vi "SV Compare Signal Configurations.vi"(5 "SV Signal 1":refnum<class "SV Signal.lvclass">, 9 "SV Signal 2":refnum<class "SV Signal.lvclass">) -> (8 "equal?":bool)   [LabVIEW 2017, in "SV Signal.lvclass"]
doc: "This VI determines if two signal configurations are equal with respect to SV Update Signal. If they are equal, it means there will be no change in the output signal after calling SV Update Signal.vi. You can use this VI to determine if it is necessary to call SV Update Signal."
uses:
  <vilib>/addons/_NISVFA/_Generation/Signal Generation/SV Signal/SV Signal.lvclass
  <vilib>/addons/_NISVFA/_Generation/Signal Generation/SV Signal/SV Signal.lvclass/SV Signal.ctl
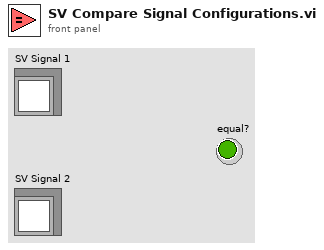
[diagram p1: front panel]
types:
  T1 = typedef "SV Signal.lvclass/sv_System Timing Model.ctl" = i64
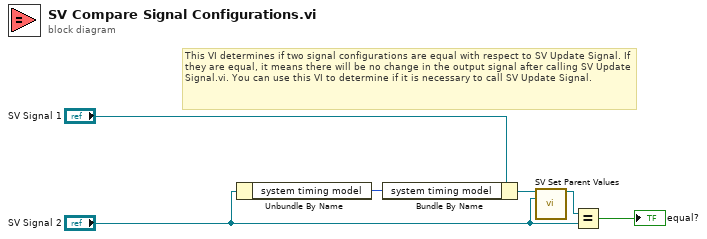
[diagram p0: block diagram]
diagram:
  # "This VI determines if two signal configurations are equal with respect to SV Update Signal. If they are equal, it means there will be no change in the output signal after calling SV Update Signal.vi. You can use this VI to determine if it is necessary to call SV Update Signal."
  n1 = Unbundle By Name("SV Signal 2") -> ("system timing model"=w2:T1)
  n2 = Bundle By Name(cluster="SV Signal 1", "system timing model"=w2) -> (w3:refnum<class "SV Signal.lvclass">)
  n3 = call-dynamic "SV Set Parent Values.vi"("child class in"=w3, "parent class"="SV Signal 2") -> ("child class out"=w1:refnum<class "SV Signal.lvclass">)  [unwired: 12 in, 1 out]
  n4 = Equal?(x=w1, y="SV Signal 2") -> (x = y?=→"equal?":bool)
